vi "超标留样通讯.vi"(8 "Error in":errorcluster caption="Error in (no error)") -> (0 "error out":errorcluster, 2 "MB session in":refnum<class "MB_Master.lvclass">)   [LabVIEW 2016, in "超标留样集成.lvlib" / "ESTD1200.lvlib"]
uses:
  ESTD1200.lvlib
  <vilib>/Plasmionique/MB Master/MB_Master/MB_Master.lvclass
  <vilib>/Plasmionique/MB Master/MB_Master_Serial/MB_Master_Serial.lvclass
  E:/Program Files (x86)/National Instruments/LabVIEW 2016/vi.lib/Plasmionique/MB Master/MB_Master/MB_Master.lvclass
  <vilib>/Plasmionique/MB Master/MB_Master_TCP/MB_Master_TCP.lvclass
  <vilib>/Plasmionique/MB Master/MB Master.lvlib
panel:
  out "布尔":bool
  in  "启用模块":bool
  in  "取样":bool
  in  "系统复位":bool
  in  "软重启":bool
  in  "开门":bool
  in  "停止采样":bool
  in  "启动采样":bool
  in  "读取传感器实时浓度":bool
  in  "读取状态告警区":bool
  in  "读取系统设置区":bool
  in  "读取采样模式区":bool
  in  "读取采样状态区":bool
  out "传感器实时浓度":T1
  out "状态告警区":T2 {"告警代码" items=["无告警", "通讯异常(采样器与工控机通讯)", "滑台电机异常(过温/过流)", "蠕动泵异常(过温/过流)", "转盘电机异常(过温/过流)", "编码器异常", "转盘原点传感器异常", "滑台原点传感器异常", "冰箱温度异常", "冰箱通讯异常", "门禁锁异常", "串口屏通讯异常", "SD卡异常告警", "Flash异常告警(W25Q32)", "留样失败", "瓶满告警", "复位异常"]; "采样模式" items=["定时采样", "外控采样", "时间等比", "流量等比", "液位等比"]; "当前进程" items=["待机", "电机复位", "采样瓶转到采样区", "采样瓶排空", "采样泵管润洗", "采样瓶再排空", "采样", "采样泵反转排空管路", "取样瓶转到取样区"]}
  out "系统设置区":T3
  out "采样模式区":T4 {"采样模式" items=["定时采样", "外控采样", "时间等比", "流量等比", "液位等比"]}
  out "采样状态区":T5 {"当前进程" items=["待机", "电机复位", "采样瓶转到采样区", "采样瓶排空", "采样泵管润洗", "采样瓶再排空", "采样", "采样泵反转排空管路", "取样瓶转到取样区"]; "采样模式" items=["定时采样", "外控采样", "时间等比", "流量等比", "液位等比"]; "采样器状态" items=["空闲", "忙碌"]}
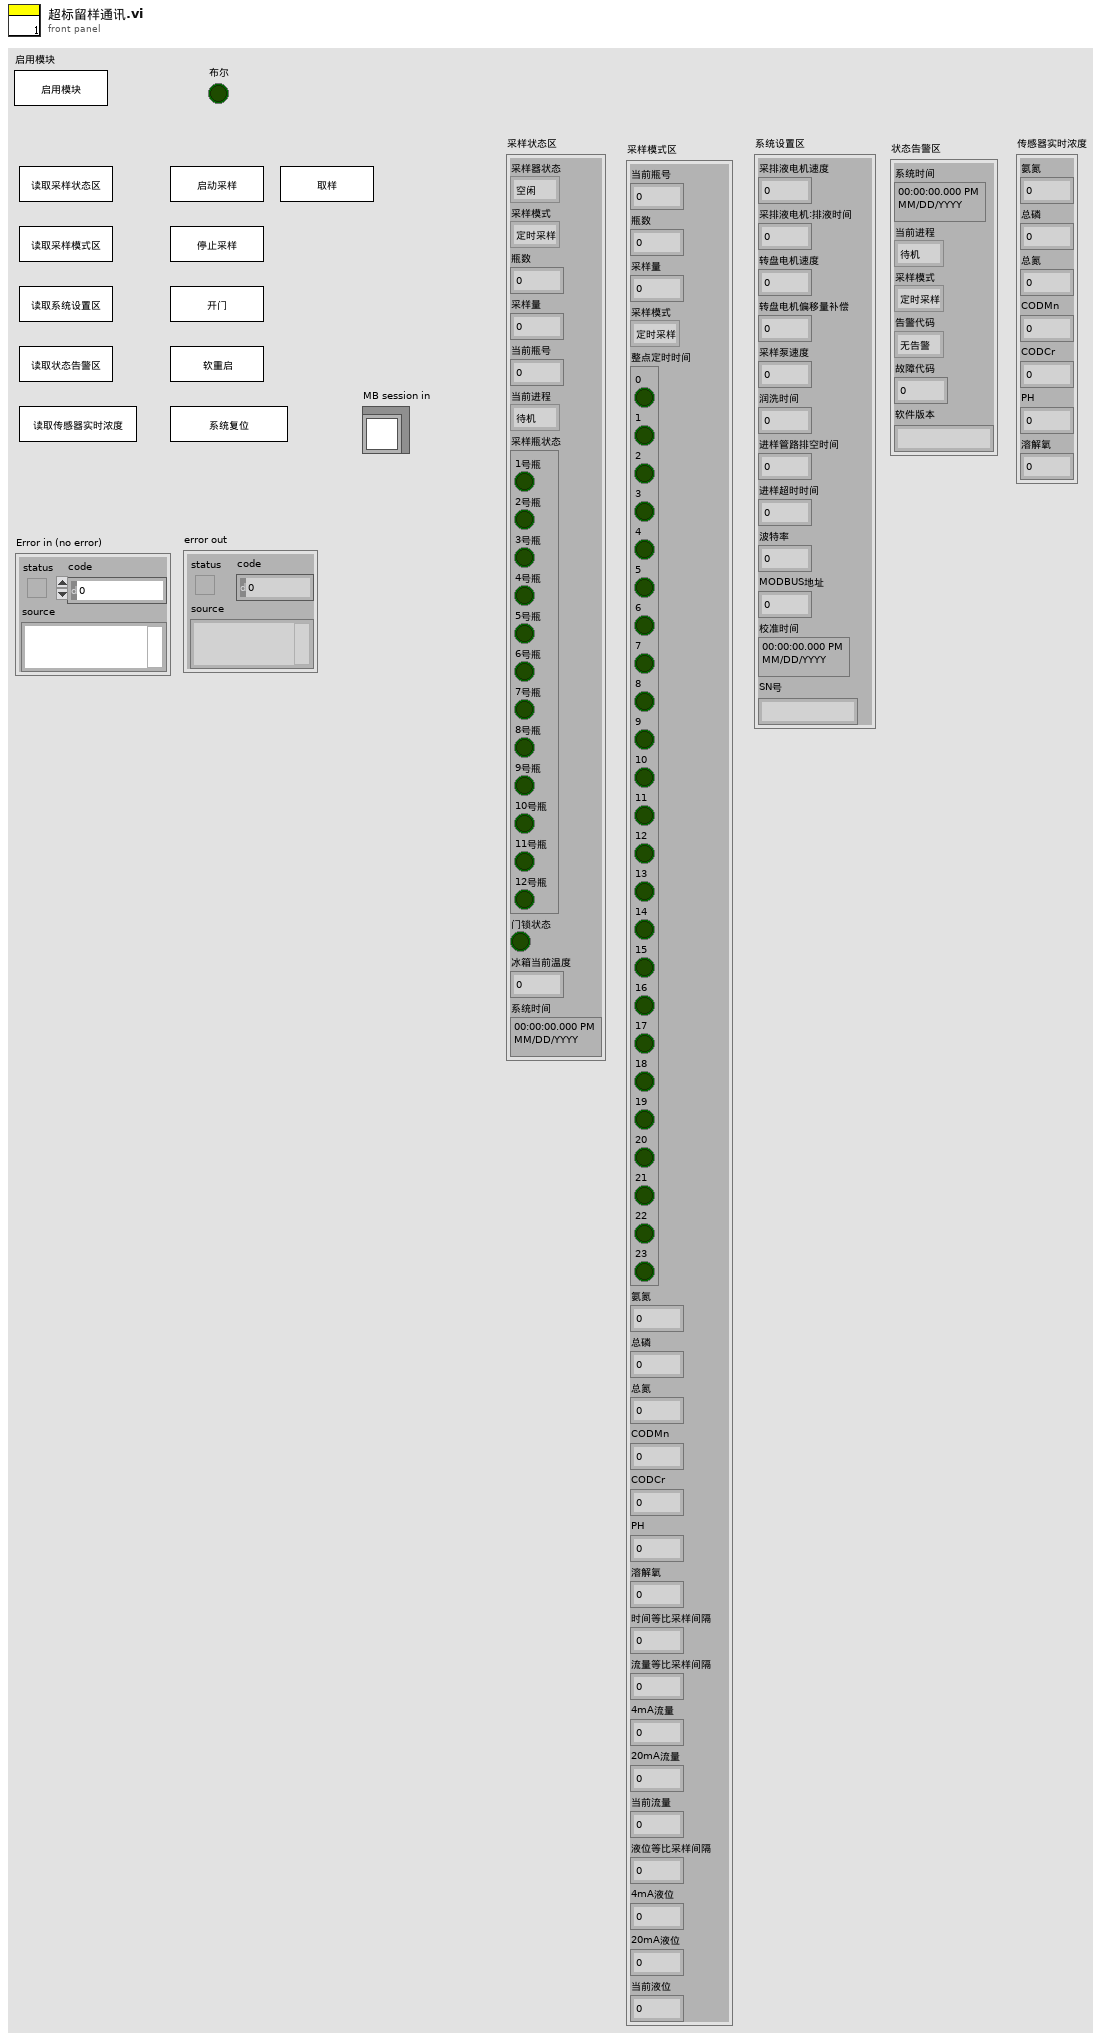
[diagram p1: front panel]
types:
  T1 = cluster{"氨氮":sgl, "总磷":sgl, "总氮":sgl, "CODMn":sgl, "CODCr":sgl, "PH":sgl, "溶解氧":sgl}
  T2 = cluster{"系统时间":timestamp, "当前进程":u16, "采样模式":u16, "告警代码":u16, "故障代码":u16, "软件版本":string}
  T3 = cluster{"采排液电机速度":u16, "采排液电机:排液时间":u16, "转盘电机速度":u16, "转盘电机偏移量补偿":u16, "采样泵速度":u16, "润洗时间":u16, "进样管路排空时间":u16, "进样超时时间":u16, "波特率":u16, "MODBUS地址":u16, "校准时间":timestamp, "SN号":string}
  T4 = cluster{"当前瓶号":u16, "瓶数":u16, "采样量":u16, "采样模式":u16, "整点定时时间":cluster{"0":bool, "1":bool, "2":bool, "3":bool, "4":bool, "5":bool, "6":bool, "7":bool, "8":bool, "9":bool, "10":bool, "11":bool, "12":bool, "13":bool, "14":bool, "15":bool, "16":bool, "17":bool, "18":bool, "19":bool, "20":bool, "21":bool, "22":bool, "23":bool}, "氨氮":sgl, "总磷":sgl, "总氮":sgl, "CODMn":sgl, "CODCr":sgl, "PH":sgl, "溶解氧":sgl, "时间等比采样间隔":u16, "流量等比采样间隔":sgl, "4mA流量":sgl, "20mA流量":sgl, "当前流量":sgl, "液位等比采样间隔":sgl, "4mA液位":sgl, "20mA液位":sgl, "当前液位":sgl}
  T5 = cluster{"采样器状态":u16, "采样模式":u16, "瓶数":u16, "采样量":u16, "当前瓶号":u16, "当前进程":u16, "采样瓶状态":cluster{"1号瓶":bool, "2号瓶":bool, "3号瓶":bool, "4号瓶":bool, "5号瓶":bool, "6号瓶":bool, "7号瓶":bool, "8号瓶":bool, "9号瓶":bool, "10号瓶":bool, "11号瓶":bool, "12号瓶":bool}, "门锁状态":bool, "冰箱当前温度":sgl, "系统时间":timestamp}
  T6 = typedef "队列data.ctl" = cluster{"命令":string, "data":cluster{"站号":u16, "控制命令":u16[]}}
  T7 = cluster{"命令":string, "data":cluster{"站号":u16, "控制命令":u16[]}}
  T8 = cluster{"baud rate (bps)":u32, "stop bits":u16, "parity":u16, "flow control":u16, "timeout":u32, "retries":i32}
  T9 = cluster{"[0]":bool, "[1]":bool, "[2]":bool, "[3]":bool, "[4]":bool, "[5]":bool, "[6]":bool, "[7]":bool, "[8]":bool, "[9]":bool, "[10]":bool, "[11]":bool}
  T10 = cluster{u16, u16, u16, u16, u16, u16, cluster{"[0]":bool, "[1]":bool, "[2]":bool, "[3]":bool, "[4]":bool, "[5]":bool, "[6]":bool, "[7]":bool, "[8]":bool, "[9]":bool, "[10]":bool, "[11]":bool}, bool, dbl, "time stamp":timestamp}
  T11 = cluster{"[0]":bool, "[1]":bool, "[2]":bool, "[3]":bool, "[4]":bool, "[5]":bool, "[6]":bool, "[7]":bool, "[8]":bool, "[9]":bool, "[10]":bool, "[11]":bool, "[12]":bool, "[13]":bool, "[14]":bool, "[15]":bool, "[16]":bool, "[17]":bool, "[18]":bool, "[19]":bool, "[20]":bool, "[21]":bool, "[22]":bool, "[23]":bool}
  T12 = cluster{u16, u16, u16, u16, cluster{"[0]":bool, "[1]":bool, "[2]":bool, "[3]":bool, "[4]":bool, "[5]":bool, "[6]":bool, "[7]":bool, "[8]":bool, "[9]":bool, "[10]":bool, "[11]":bool, "[12]":bool, "[13]":bool, "[14]":bool, "[15]":bool, "[16]":bool, "[17]":bool, "[18]":bool, "[19]":bool, "[20]":bool, "[21]":bool, "[22]":bool, "[23]":bool}, sgl, sgl, sgl, sgl, sgl, sgl, sgl, u16, sgl, sgl, sgl, sgl, sgl, sgl, sgl, sgl}
  T13 = cluster{u16, u16, u16, u16, u16, u16, u16, u16, u16, u16, "time stamp":timestamp, string}
  T14 = cluster{"time stamp":timestamp, u16, u16, u16, u16, string}
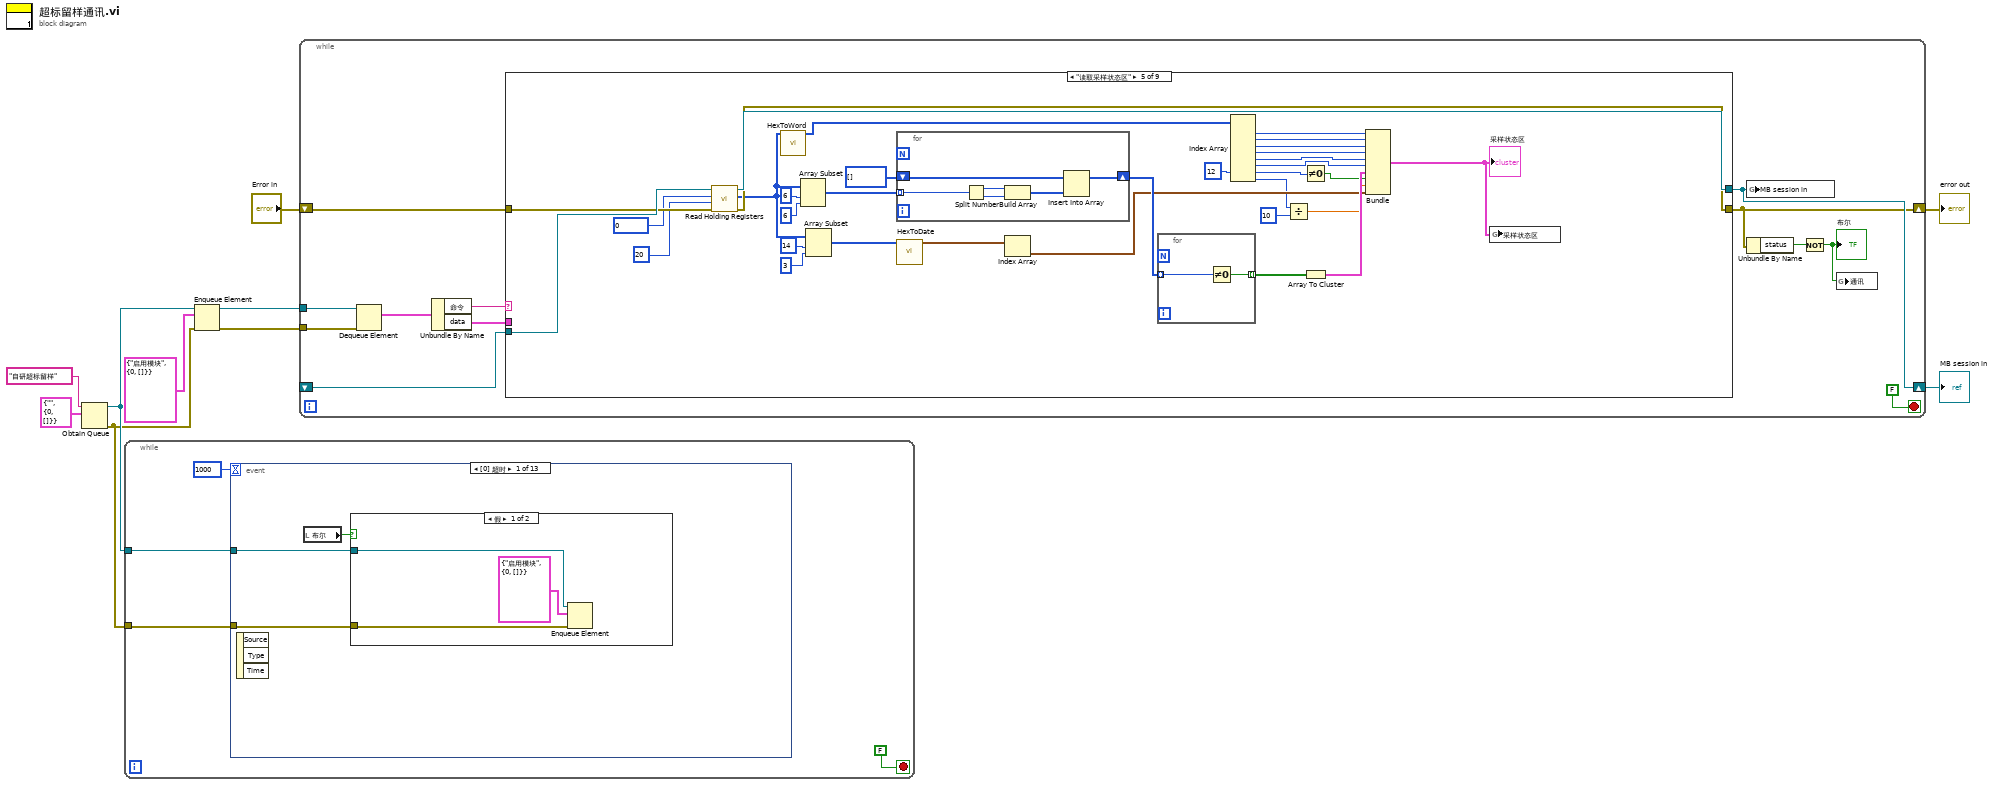
[diagram p0: block diagram]
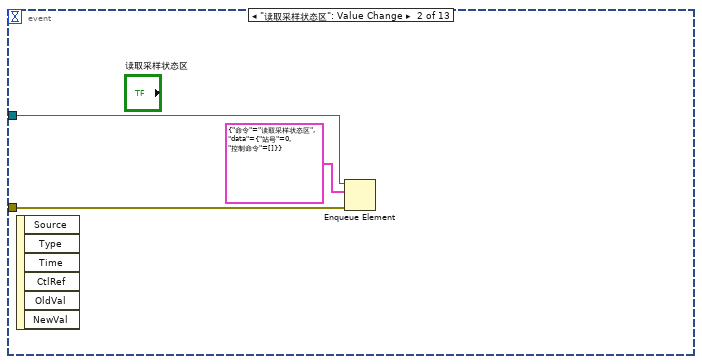
[diagram p3: hidden frame]
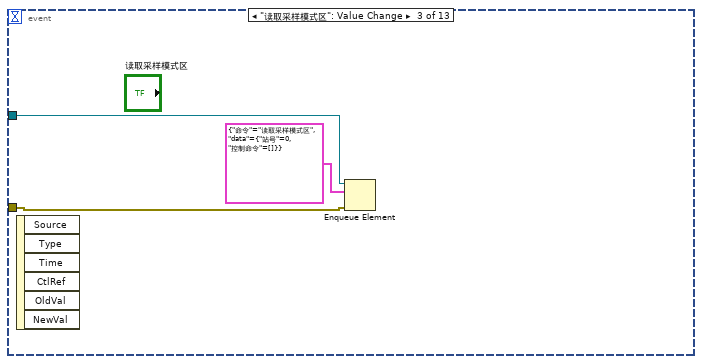
[diagram p4: hidden frame]
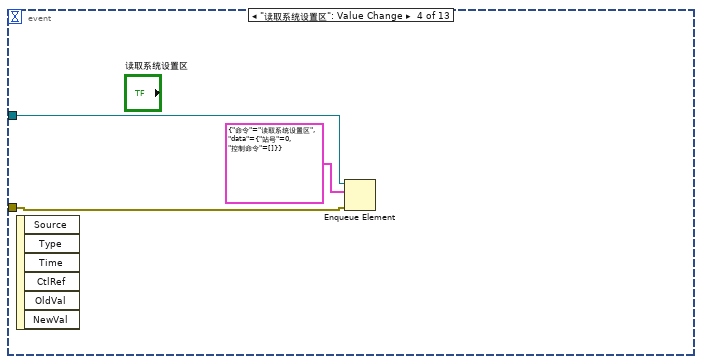
[diagram p5: hidden frame]
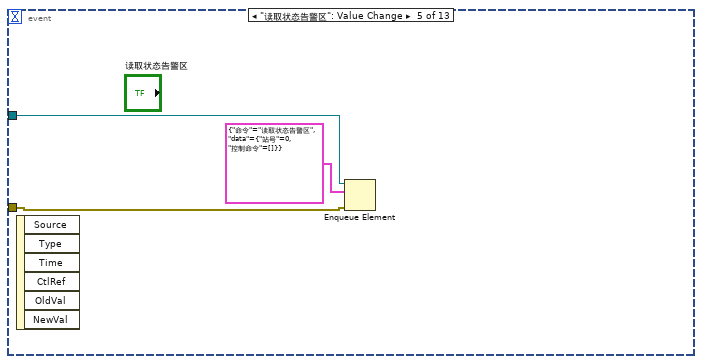
[diagram p6: hidden frame]
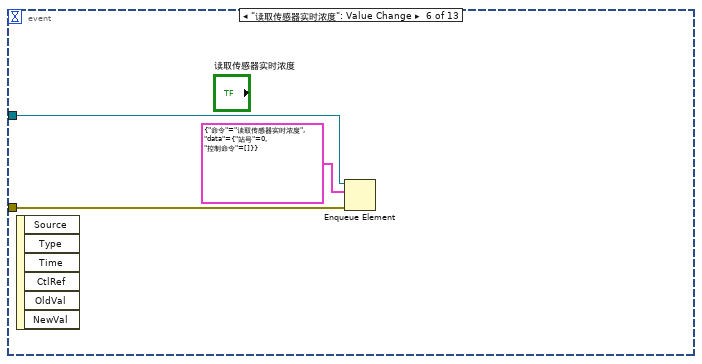
[diagram p7: hidden frame]
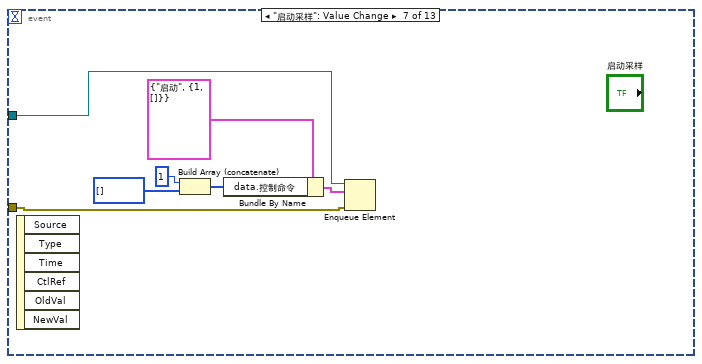
[diagram p8: hidden frame]
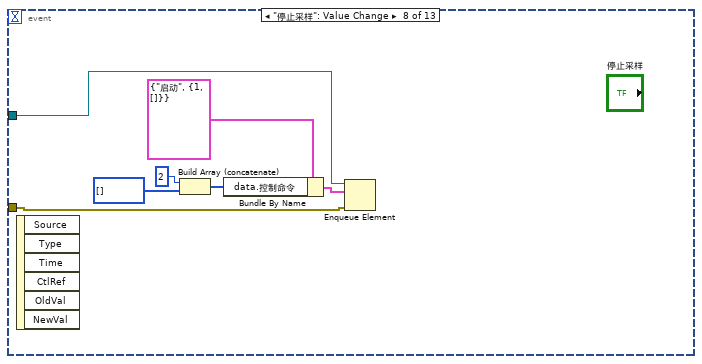
[diagram p9: hidden frame]
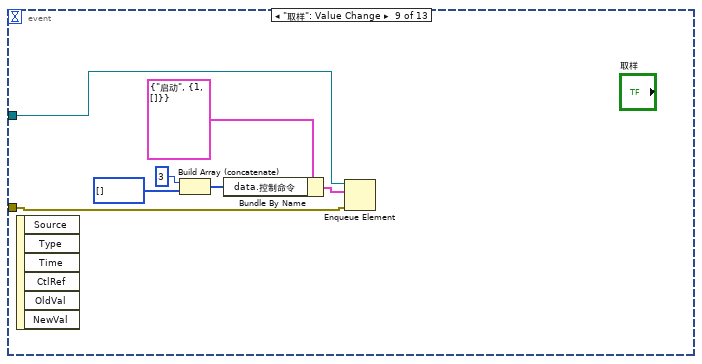
[diagram p10: hidden frame]
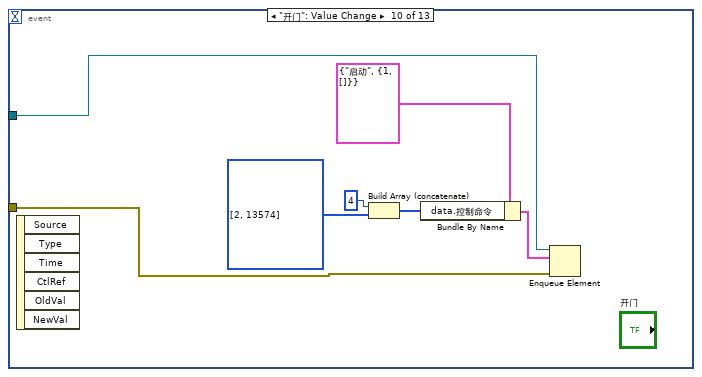
[diagram p11: hidden frame]
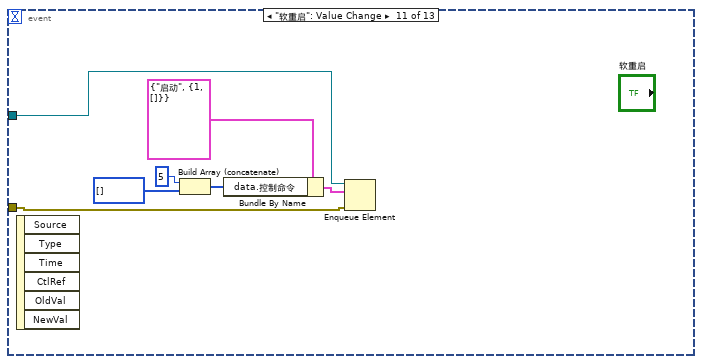
[diagram p12: hidden frame]
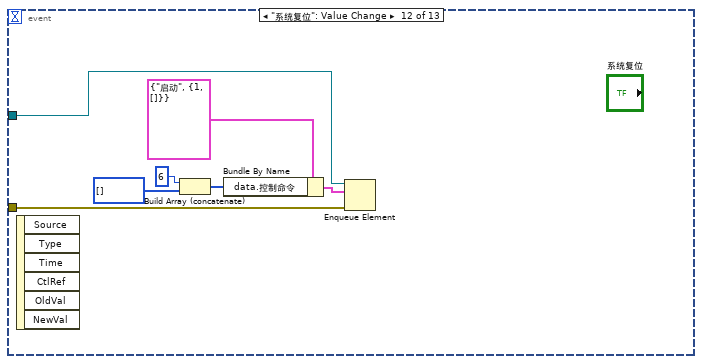
[diagram p13: hidden frame]
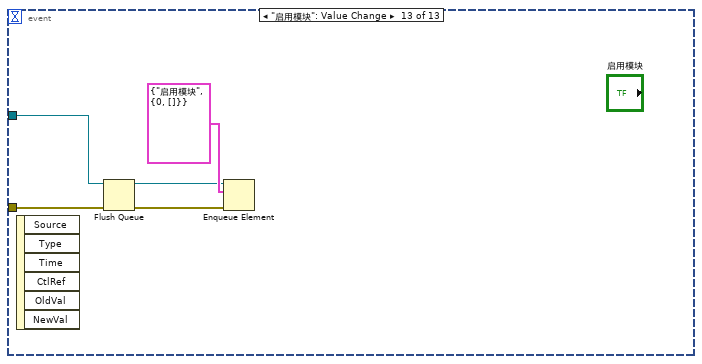
[diagram p14: hidden frame]
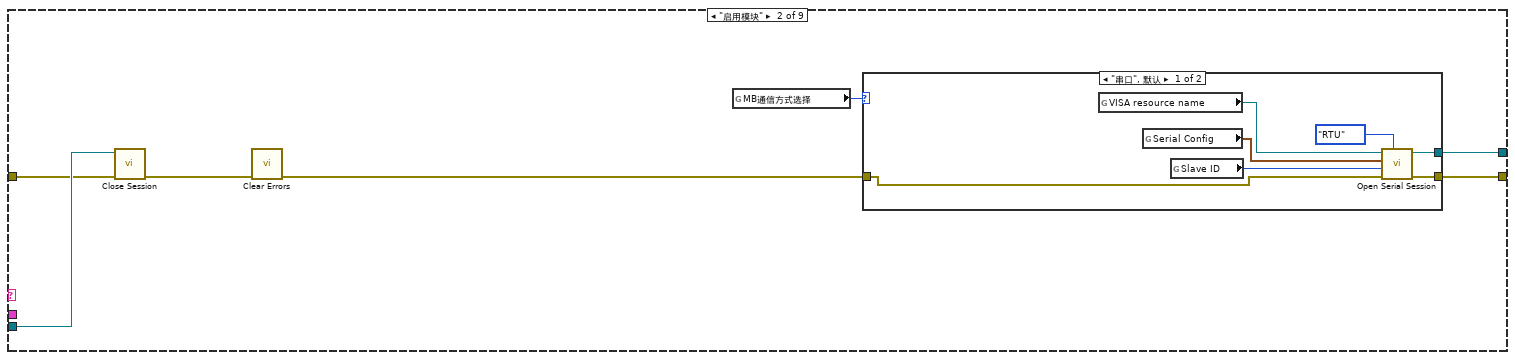
[diagram p16: hidden frame]
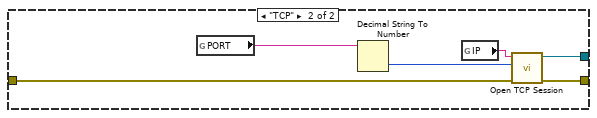
[diagram p17: hidden frame]
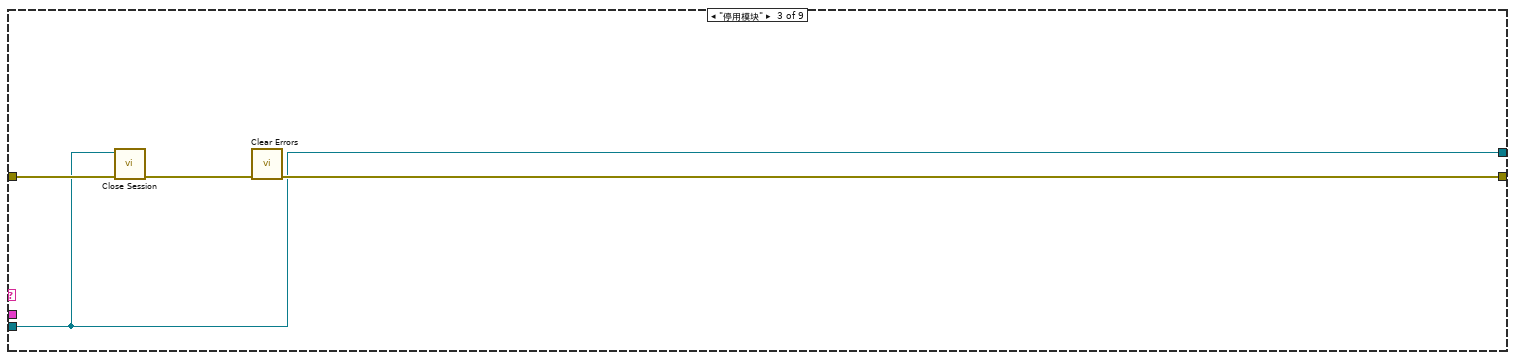
[diagram p18: hidden frame]
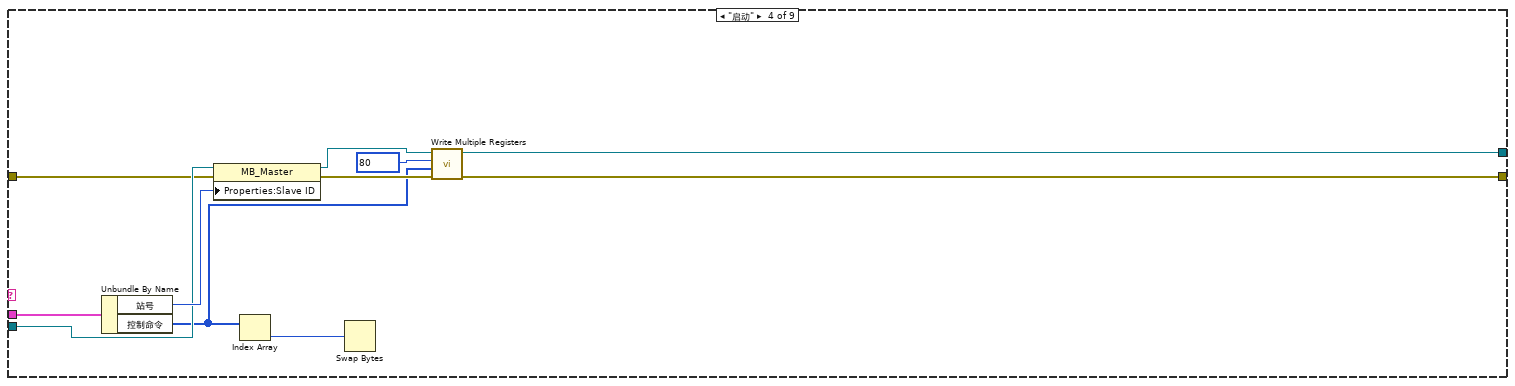
[diagram p19: hidden frame]
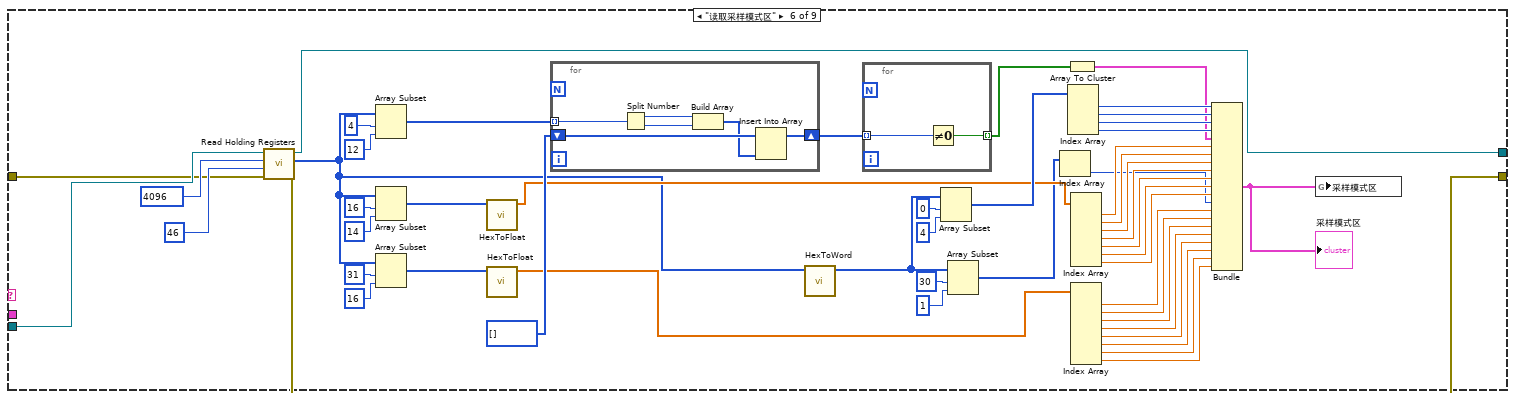
[diagram p20: hidden frame]
diagram:
  n1 = Obtain Queue(name (unnamed)="自研超标留样" ("名称（未命名）"), element data type=T6 {"命令"="", "data"={"站号"=0, "控制命令"=[]}}) -> (queue out=w5:refnum<queue>, error out=w4:errorcluster)  [unwired: 3 in, 1 out]
  n2 = while {
    tunnel: w5 -> [w13]
    tunnel: w4 -> [w12]
    stop <- FALSE stop-if-true
    n3 = event shown="[0] 超时" {
      selector: _ -> [_ _ _ _ _ _ _ _ _ _ _ _ _]
      dyn-events: _ -> [_ _ _ _ _ _ _ _ _ _ _ _ _]
      timeout: 1000 -> [_ _ _ _ _ _ _ _ _ _ _ _ _]
      tunnel: w13 -> [w16 w23 w25 w28 w31 w34 w42 w45 w52 w59 w66 w73 w81]
      tunnel: w12 -> [w15 w22 w24 w27 w30 w33 w41 w44 w51 w58 w65 w72 w79]
      event Timeout {
        n4 = event-data() -> ()  [unwired: 1 in, 3 out]
        n5 = local read "布尔"() -> (w17:bool)
        n6 = case shown="假" w17 {
          tunnel: w16 -> [w20 _]
          tunnel: w15 -> [w19 _]
          frame False {
            n7 = Enqueue Element(queue=w20, element=T7 {"命令"="启用模块", "data"={"站号"=0, "控制命令"=[]}} ("元素"), error in (no error)=w19) -> ()  [unwired: 1 in, 3 out]
          }
          frame True {
          }
        }
      }
      event "读取采样状态区": Value Change {
        n8 = event-data() -> ()  [unwired: 1 in, 6 out]
        n9 = Enqueue Element(queue=w23, element=T7 {"命令"="读取采样状态区", "data"={"站号"=0, "控制命令"=[]}} ("元素"), error in (no error)=w22) -> ()  [unwired: 1 in, 3 out]
      }
      event "读取采样模式区": Value Change {
        n10 = event-data() -> ()  [unwired: 1 in, 6 out]
        n11 = Enqueue Element(queue=w25, element=T7 {"命令"="读取采样模式区", "data"={"站号"=0, "控制命令"=[]}} ("元素"), error in (no error)=w24) -> ()  [unwired: 1 in, 3 out]
      }
      event "读取系统设置区": Value Change {
        n12 = event-data() -> ()  [unwired: 1 in, 6 out]
        n13 = Enqueue Element(queue=w28, element=T7 {"命令"="读取系统设置区", "data"={"站号"=0, "控制命令"=[]}} ("元素"), error in (no error)=w27) -> ()  [unwired: 1 in, 3 out]
      }
      event "读取状态告警区": Value Change {
        n14 = event-data() -> ()  [unwired: 1 in, 6 out]
        n15 = Enqueue Element(queue=w31, element=T7 {"命令"="读取状态告警区", "data"={"站号"=0, "控制命令"=[]}} ("元素"), error in (no error)=w30) -> ()  [unwired: 1 in, 3 out]
      }
      event "读取传感器实时浓度": Value Change {
        n16 = event-data() -> ()  [unwired: 1 in, 6 out]
        n17 = Enqueue Element(queue=w34, element=T7 {"命令"="读取传感器实时浓度", "data"={"站号"=0, "控制命令"=[]}} ("元素"), error in (no error)=w33) -> ()  [unwired: 1 in, 3 out]
      }
      event "启动采样": Value Change {
        n18 = event-data() -> ()  [unwired: 1 in, 6 out]
        n19 = Build Array (concatenate)(u16 1 ("数值"), u16[] [] ("控制命令")) -> (w38:u16[])
        n20 = Bundle By Name(cluster=T7 {"命令"="启动", "data"={"站号"=1, "控制命令"=[]}} ("元素"), "data.控制命令"=w38) -> (w37:T7)
        n21 = Enqueue Element(queue=w42, element=w37, error in (no error)=w41) -> ()  [unwired: 1 in, 3 out]
      }
      event "停止采样": Value Change {
        n22 = event-data() -> ()  [unwired: 1 in, 6 out]
        n23 = Build Array (concatenate)(u16 2 ("数值"), u16[] [] ("控制命令")) -> (w47:u16[])
        n24 = Bundle By Name(cluster=T7 {"命令"="启动", "data"={"站号"=1, "控制命令"=[]}} ("元素"), "data.控制命令"=w47) -> (w46:T7)
        n25 = Enqueue Element(queue=w45, element=w46, error in (no error)=w44) -> ()  [unwired: 1 in, 3 out]
      }
      event "取样": Value Change {
        n26 = event-data() -> ()  [unwired: 1 in, 6 out]
        n27 = Build Array (concatenate)(u16 3 ("数值"), u16[] [] ("控制命令")) -> (w54:u16[])
        n28 = Bundle By Name(cluster=T7 {"命令"="启动", "data"={"站号"=1, "控制命令"=[]}} ("元素"), "data.控制命令"=w54) -> (w53:T7)
        n29 = Enqueue Element(queue=w52, element=w53, error in (no error)=w51) -> ()  [unwired: 1 in, 3 out]
      }
      event "开门": Value Change {
        n30 = event-data() -> ()  [unwired: 1 in, 6 out]
        n31 = Build Array (concatenate)(u16 4 ("数值"), u16[] [2, 13574] ("控制命令")) -> (w61:u16[])
        n32 = Bundle By Name(cluster=T7 {"命令"="启动", "data"={"站号"=1, "控制命令"=[]}} ("元素"), "data.控制命令"=w61) -> (w60:T7)
        n33 = Enqueue Element(queue=w59, element=w60, error in (no error)=w58) -> ()  [unwired: 1 in, 3 out]
      }
      event "软重启": Value Change {
        n34 = event-data() -> ()  [unwired: 1 in, 6 out]
        n35 = Build Array (concatenate)(u16 5 ("数值"), u16[] [] ("控制命令")) -> (w68:u16[])
        n36 = Bundle By Name(cluster=T7 {"命令"="启动", "data"={"站号"=1, "控制命令"=[]}} ("元素"), "data.控制命令"=w68) -> (w67:T7)
        n37 = Enqueue Element(queue=w66, element=w67, error in (no error)=w65) -> ()  [unwired: 1 in, 3 out]
      }
      event "系统复位": Value Change {
        n38 = event-data() -> ()  [unwired: 1 in, 6 out]
        n39 = Build Array (concatenate)(u16 6 ("数值"), u16[] [] ("控制命令")) -> (w75:u16[])
        n40 = Bundle By Name(cluster=T7 {"命令"="启动", "data"={"站号"=1, "控制命令"=[]}} ("元素"), "data.控制命令"=w75) -> (w74:T7)
        n41 = Enqueue Element(queue=w73, element=w74, error in (no error)=w72) -> ()  [unwired: 1 in, 3 out]
      }
      event "启用模块": Value Change {
        n42 = event-data() -> ()  [unwired: 1 in, 6 out]
        n43 = Flush Queue(queue=w81, error in (no error)=w79) -> (queue out=w80:refnum<queue>, error out=w78:errorcluster)  [unwired: 1 out]
        n44 = Enqueue Element(queue=w80, element=T7 {"命令"="启用模块", "data"={"站号"=0, "控制命令"=[]}} ("元素"), error in (no error)=w78) -> ()  [unwired: 1 in, 3 out]
      }
    }
  }
  n45 = Enqueue Element(queue=w5, element=T7 {"命令"="启用模块", "data"={"站号"=0, "控制命令"=[]}} ("元素"), error in (no error)=w4) -> (queue out=w3:refnum<queue>, error out=w2:errorcluster)  [unwired: 1 in, 1 out]
  n46 = while {
    tunnel: w3 -> [w94]
    tunnel: w2 -> [w93]
    shift-right: [w89] -> w7
    shift-left: _ -> [w92]
    shift-right: [w84] -> w8
    shift-left: "Error in" -> [w91]
    stop <- FALSE stop-if-true
    n47 = Dequeue Element(queue=w94, error in (no error)=w93) -> (element=w88:T6)  [unwired: 1 in, 3 out]
    n48 = Unbundle By Name(w88) -> ("命令"=w87:string, "data"=w86:cluster{"站号":u16, "控制命令":u16[]})
    n49 = case shown="\"读取采样状态区\"" w87 {
      tunnel: [w96 w100 w117 w122 w162 w216 w233 w276 w314] -> w89
      tunnel: w92 -> [w96 w99 w117 w125 w164 w220 w259 w301 w317]
      tunnel: [w95 w98 w118 w121 w161 w215 w232 w275 w313] -> w84
      tunnel: w91 -> [w95 w97 w119 w124 w163 w219 w258 w300 w316]
      tunnel: w86 -> [_ _ _ w131 _ _ _ _ _]
      frame "", Default {
      }
      frame "启用模块" {
        n50 = call-dynamic "Close Session.vi"("error in (no error)"=w97, "MB session in"=w99) -> ("error out"=w103:errorcluster)  [unwired: 9 in]
        n51 = call <vilib>:"Clear Errors.vi"("error in (no error)"=w103) -> ("error out"=w102:errorcluster)  [unwired: 5 in, 1 out]
        n52 = global read "串口参数断电保存全局变量.vi" "MB通信方式选择"() -> (w101:enum16{"串口", "TCP"})
        n53 = case shown="\"串口\", 默认" w101 {
          tunnel: [w109 w115] -> w98
          tunnel: [w104 w113] -> w100
          tunnel: w102 -> [w108 w114]
          frame "串口", Default {
            n54 = global read "串口参数断电保存全局变量.vi" "VISA resource name"() -> (w107:refnum<visa-resource-name>)
            n55 = global read "串口参数断电保存全局变量.vi" "Serial Config"() -> (w105:T8)
            n56 = global read "串口参数断电保存全局变量.vi" "Slave ID"() -> (w106:u8)
            n57 = call <vilib>:"Open Serial Session.vi"("Mode (RTU)"=enum16{"RTU", "ASCII"}."RTU", "Error in"=w108, "Slave ID"=w106, "Serial Config"=w105, "VISA Resource"=w107) -> ("Error out"=w109:errorcluster, "MB_Serial session"=w104:refnum<class "MB_Master_Serial.lvclass">)  [unwired: 5 in]
          }
          frame "TCP" {
            n58 = global read "串口参数断电保存全局变量.vi" "PORT"() -> (w111:string)
            n59 = Decimal String To Number(string=w111) -> (number=w116:i32)  [unwired: 2 in, 1 out]
            n60 = global read "串口参数断电保存全局变量.vi" "IP"() -> (w112:string)
            n61 = call <vilib>:"Open TCP Session.vi"("error in (no error)"=w114, "Port (502)"=w116, "IP Address"=w112) -> ("error out"=w115:errorcluster, "MB_TCP session"=w113:refnum<class "MB_Master_TCP.lvclass">)  [unwired: 7 in]
          }
        }
      }
      frame "停用模块" {
        n62 = call-dynamic "Close Session.vi"("error in (no error)"=w119, "MB session in"=w117) -> ("error out"=w120:errorcluster)  [unwired: 9 in]
        n63 = call <vilib>:"Clear Errors.vi"("error in (no error)"=w120) -> ("error out"=w118:errorcluster)  [unwired: 5 in, 1 out]
      }
      frame "启动" {
        n64 = Unbundle By Name(w131) -> ("站号"=w126:u16, "控制命令"=w123:u16[])
        n65 = property class="MB_Master"(reference=w125, error in=w124, "Properties:Slave ID"=w126) -> (reference out=w128:refnum<class "MB_Master.lvclass">, error out=w127:errorcluster)
        n66 = Index Array(array=w123) -> (element=w130:u16)  [unwired: 1 in]
        n67 = Swap Bytes(anything=w130) -> ()  [unwired: 1 out]
        n68 = call <vilib>:"Write Multiple Registers.vi"("error in (no error)"=w127, "values"=w123, "starting address"=u16 80, "MB session in"=w128) -> ("error out"=w121:errorcluster, "MB session out"=w122:refnum<class "MB_Master.lvclass">)  [unwired: 6 in]
      }
      frame "读取采样状态区" {
        n69 = call <vilib>:"Read Holding Registers.vi"("error in (no error)"=w163, "quantity"=u16 20, "starting address"=u16 0, "MB session in"=w164) -> ("error out"=w161:errorcluster, "Registers"=w135:u16[], "MB session out"=w162:refnum<class "MB_Master.lvclass">)  [unwired: 5 in]
        n70 = call "HexToWord.vi"("Registers"=w135) -> ("数组"=w152:u16[])  [unwired: 10 in]
        n71 = Array Subset(array=w135, index=6 ("索引"), length=6 ("长度")) -> (w146:u16[])
        n72 = Array Subset(array=w135, index=14 ("索引"), length=3 ("长度")) -> (w139:u16[])
        n73 = for {
          tunnel: w146 -> [w172] mode=indexing
          shift-right: [w168] -> w148
          shift-left: u8[] [] -> [w169]
          n74 = Split Number(x=w172) -> (hi(x)=w171:u8, lo(x)=w170:u8)
          n75 = Build Array(w171, w170) -> (w167:u8[])
          n76 = Insert Into Array(array=w169, new element=w167) -> (w168:u8[])  [unwired: 1 in]
        }
        n77 = call "HexToDate.vi"("数组输入"=w139) -> ("数组输出"=w138:timestamp[])  [unwired: 10 in]
        n78 = Index Array(array=w138) -> (element=w137:timestamp)  [unwired: 1 in]
        n79 = for {
          tunnel: w148 -> [w166] mode=indexing
          tunnel: [w165] -> w147 mode=indexing
          n80 = Not Equal To 0?(x=w166) -> (x != 0?=w165:bool)
        }
        n81 = Index Array(array=w152, index #7=12 ("索引")) -> (element #1=w158:u16, element #2=w157:u16, element #3=w156:u16, element #4=w155:u16, element #5=w154:u16, element #6=w153:u16, element #7=w143:u16, element #8=w134:u16)  [unwired: 7 in]
        n82 = Divide(x=w134, y=u16 10) -> (x/y=w132:dbl)
        n83 = Not Equal To 0?(x=w143) -> (x != 0?=w142:bool)
        n84 = Array To Cluster(array=w147) -> (cluster=w145:T9)
        n85 = Bundle(w158, w157, w156, w155, w154, w153, w145, w142, w132, "time stamp"=w137) -> (w136:T10)  [unwired: 1 in]
        "采样状态区" <- w136
        n86 = global write "超标留样全局.vi" "采样状态区"(w136) -> ()
      }
      frame "读取采样模式区" {
        n87 = call <vilib>:"Read Holding Registers.vi"("error in (no error)"=w219, "quantity"=u16 46, "starting address"=u16 4096, "MB session in"=w220) -> ("error out"=w215:errorcluster, "Registers"=w174:u16[], "MB session out"=w216:refnum<class "MB_Master.lvclass">)  [unwired: 5 in]
        n88 = Array Subset(array=w174, index=4 ("索引"), length=12 ("长度")) -> (w205:u16[])
        n89 = Array Subset(array=w174, index=16 ("索引"), length=14 ("长度")) -> (w200:u16[])
        n90 = Array Subset(array=w174, index=31 ("索引"), length=16 ("长度")) -> (w187:u16[])
        n91 = call "HexToFloat.vi"("数组输入"=w200) -> ("数组输出"=w199:sgl[])  [unwired: 10 in]
        n92 = call "HexToFloat.vi"("数组输入"=w187) -> ("数组输出"=w184:sgl[])  [unwired: 10 in]
        n93 = for {
          tunnel: w205 -> [w230] mode=indexing
          shift-right: [w226] -> w209
          shift-left: u8[] [] -> [w227]
          n94 = Split Number(x=w230) -> (hi(x)=w229:u8, lo(x)=w228:u8)
          n95 = Build Array(w229, w228) -> (w225:u8[])
          n96 = Insert Into Array(array=w227, new element=w225) -> (w226:u8[])  [unwired: 1 in]
        }
        n97 = call "HexToWord.vi"("Registers"=w174) -> ("数组"=w173:u16[])  [unwired: 10 in]
        n98 = for {
          tunnel: w209 -> [w224] mode=indexing
          tunnel: [w223] -> w204 mode=indexing
          n99 = Not Equal To 0?(x=w224) -> (x != 0?=w223:bool)
        }
        n100 = Array Subset(array=w173, index=0 ("索引"), length=4 ("长度")) -> (w208:u16[])
        n101 = Array Subset(array=w173, index=30 ("索引"), length=1 ("长度")) -> (w189:u16[])
        n102 = Index Array(array=w189) -> (element=w188:u16)  [unwired: 1 in]
        n103 = Array To Cluster(array=w204) -> (cluster=w203:T11)
        n104 = Index Array(array=w208) -> (element #1=w214:u16, element #2=w213:u16, element #3=w212:u16, element #4=w211:u16)  [unwired: 4 in]
        n105 = Index Array(array=w199) -> (element #1=w198:sgl, element #2=w197:sgl, element #3=w196:sgl, element #4=w195:sgl, element #5=w194:sgl, element #6=w193:sgl, element #7=w192:sgl)  [unwired: 7 in]
        n106 = Index Array(array=w184) -> (element #1=w183:sgl, element #2=w182:sgl, element #3=w181:sgl, element #4=w180:sgl, element #5=w179:sgl, element #6=w178:sgl, element #7=w177:sgl, element #8=w176:sgl)  [unwired: 8 in]
        n107 = Bundle(w214, w213, w212, w211, w203, w198, w197, w196, w195, w194, w193, w192, w188, w183, w182, w181, w180, w179, w178, w177, w176) -> (w175:T12)  [unwired: 1 in]
        "采样模式区" <- w175
        n108 = global write "超标留样全局.vi" "采样模式区"(w175) -> ()
      }
      frame "读取系统设置区" {
        n109 = call <vilib>:"Read Holding Registers.vi"("error in (no error)"=w258, "quantity"=u16 18, "starting address"=u16 4143, "MB session in"=w259) -> ("error out"=w232:errorcluster, "Registers"=w237:u16[], "MB session out"=w233:refnum<class "MB_Master.lvclass">)  [unwired: 5 in]
        n110 = call "HexToWord.vi"("Registers"=w237) -> ("数组"=w257:u16[])  [unwired: 10 in]
        n111 = Array Subset(array=w237, index=10 ("索引"), length=3 ("长度")) -> (w244:u16[])
        n112 = Array Subset(array=w237, index=13 ("索引"), length=6 ("长度")) -> (w238:u16[])
        n113 = call "HexToDate.vi"("数组输入"=w244) -> ("数组输出"=w243:timestamp[])  [unwired: 10 in]
        n114 = for {
          tunnel: w238 -> [w271] mode=indexing
          shift-right: [w267] -> w236
          shift-left: u8[] [] -> [w268]
          n115 = Split Number(x=w271) -> (hi(x)=w270:u8, lo(x)=w269:u8)
          n116 = Build Array(w270, w269) -> (w266:u8[])
          n117 = Insert Into Array(array=w268, new element=w266) -> (w267:u8[])  [unwired: 1 in]
        }
        n118 = Index Array(array=w243) -> (element=w242:timestamp)  [unwired: 1 in]
        n119 = for {
          tunnel: w236 -> [w265] mode=indexing
          shift-right: [w262] -> w234
          shift-left: "" -> [w263]
          n120 = Number To Decimal String(number=w265) -> (decimal integer string=w264:string)  [unwired: 1 in]
          n121 = Concatenate Strings(w263, w264) -> (w262:string)
        }
        n122 = Index Array(array=w257) -> (element #1=w256:u16, element #2=w255:u16, element #3=w254:u16, element #4=w253:u16, element #5=w252:u16, element #6=w251:u16, element #7=w250:u16, element #8=w249:u16, element #9=w248:u16, element #10=w247:u16)  [unwired: 10 in]
        n123 = Bundle(w256, w255, w254, w253, w252, w251, w250, w249, w248, w247, "time stamp"=w242, w234) -> (w231:T13)  [unwired: 1 in]
        "系统设置区" <- w231
        n124 = global write "超标留样全局.vi" "系统设置区"(w231) -> ()
      }
      frame "读取状态告警区" {
        n125 = call <vilib>:"Read Holding Registers.vi"("error in (no error)"=w300, "quantity"=u16 14, "starting address"=u16 4224, "MB session in"=w301) -> ("error out"=w277:errorcluster, "Registers"=w285:u16[], "MB session out"=w278:refnum<class "MB_Master.lvclass">)  [unwired: 5 in]
        n126 = call "HexToWord.vi"("Registers"=w285) -> ("数组"=w292:u16[])  [unwired: 10 in]
        n127 = Array Subset(array=w285, index=0 ("索引"), length=3 ("长度")) -> (w297:u16[])
        n128 = Array Subset(array=w285, index=7 ("索引"), length=8 ("长度")) -> (w284:u16[])
        n129 = call "HexToDate.vi"("数组输入"=w297) -> ("数组输出"=w296:timestamp[])  [unwired: 10 in]
        n130 = call "HexToString.vi"("数组输入"=w284) -> ("数组输出"=w283:string[])  [unwired: 10 in]
        n131 = call <vilib>:"Read Holding Registers.vi"("error in (no error)"=w277, "quantity"=u16 1, "starting address"=u16 17, "MB session in"=w278) -> ("error out"=w275:errorcluster, "Registers"=w274:u16[], "MB session out"=w276:refnum<class "MB_Master.lvclass">)  [unwired: 5 in]
        n132 = call "HexToWord.vi"("Registers"=w274) -> ("数组"=w273:u16[])  [unwired: 10 in]
        n133 = Index Array(array=w296) -> (element=w295:timestamp)  [unwired: 1 in]
        n134 = Array Subset(array=w292, index=3 ("索引"), length=4 ("长度")) -> (w291:u16[])
        n135 = Index Array(array=w291) -> (element #1=w290:u16, element #2=w289:u16, element #4=w288:u16)  [unwired: 4 in, 1 out]
        n136 = Index Array(array=w283) -> (element=w282:string)  [unwired: 1 in]
        n137 = Index Array(array=w273) -> (element=w272:u16)  [unwired: 1 in]
        n138 = Bundle("time stamp"=w295, w290, w289, w272, w288, w282) -> (w281:T14)  [unwired: 1 in]
        "状态告警区" <- w281
        n139 = global write "超标留样全局.vi" "状态告警区"(w281) -> ()
      }
      frame "读取传感器实时浓度" {
        n140 = call <vilib>:"Read Holding Registers.vi"("error in (no error)"=w316, "quantity"=u16 14, "starting address"=u16 128, "MB session in"=w317) -> ("error out"=w313:errorcluster, "Registers"=w315:u16[], "MB session out"=w314:refnum<class "MB_Master.lvclass">)  [unwired: 5 in]
        n141 = call "HexToFloat.vi"("数组输入"=w315) -> ("数组输出"=w312:sgl[])  [unwired: 10 in]
        n142 = Index Array(array=w312) -> (element #1=w311:sgl, element #2=w310:sgl, element #3=w309:sgl, element #4=w308:sgl, element #5=w307:sgl, element #6=w306:sgl, element #7=w305:sgl)  [unwired: 7 in]
        n143 = Bundle(w311, w310, w309, w308, w307, w306, w305) -> (w304:cluster{sgl, sgl, sgl, sgl, sgl, sgl, sgl})  [unwired: 1 in]
        "传感器实时浓度" <- w304
        n144 = global write "超标留样全局.vi" "传感器实时浓度"(w304) -> ()
      }
    }
    n145 = global write "超标留样全局.vi" "MB session in"(w89) -> ()
    n146 = Unbundle By Name(w84) -> ("status"=w85:bool)
    n147 = Not(x=w85) -> (.not. x?=w83:bool)
    "布尔" <- w83
    n148 = global write "超标留样全局.vi" "通讯"(w83) -> ()
  }
  "error out" <- w8
  "MB session in" <- w7
